vi "RSZVB Set Fixed Power To Signal.vi"(7 "Fixed Power (-25.0)":dbl=-25.0 format="%^.3e", 8 "error in (no error)":errorcluster {"code" format="%.0x"}, 9 "Signal (RF)":i32(ring) items=["RF"=0, "IF"=2, "LO 1"=3, "LO 2"=4, "Aux LO"=5], 10 "Channel (1)":i32=1, 11 "VISA resource name":refnum<visa-resource-name>) -> (0 "error out":errorcluster {"code" format="%.0x"}, 3 "VISA resource name out":refnum<visa-resource-name>)   [LabVIEW 2011]
doc: "This VI assigns a fixed power to the RF, LO 1, LO 2, Aux LO, or to the IF signal.\n\nRemote-control command(s):\nSOURce<Ch>:FREQuency<Pt>:CONVersion:MIXer:PMFixed RF | LO | LO1 | LO2 | AUXLo | IF, <fixed_power>"
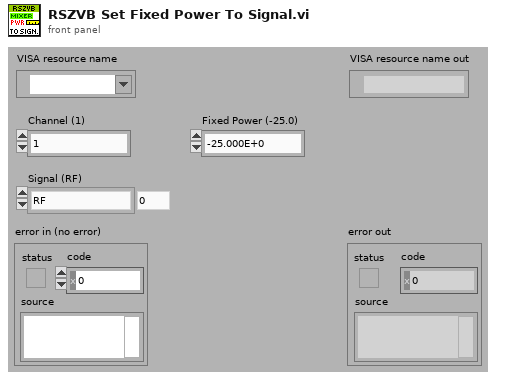
[diagram p1: front panel]
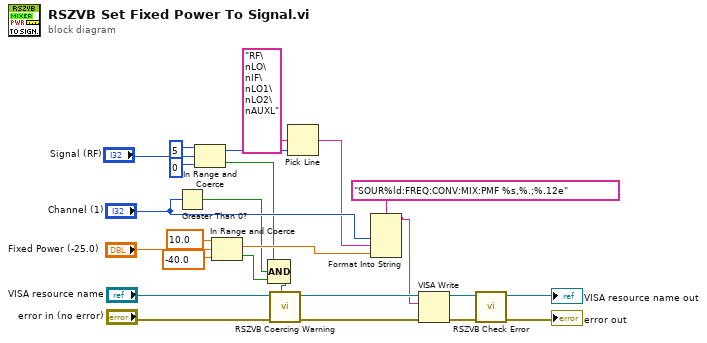
[diagram p0: block diagram]
diagram:
  n1 = Greater Than 0?(x="Channel (1)") -> (x > 0?=w4:bool)
  n2 = In Range and Coerce(upper limit=5, x="Signal (RF)", lower limit=0) -> (coerced(x)=w8:i32, In Range?=w1:bool)
  n3 = In Range and Coerce(upper limit=10.0, x="Fixed Power (-25.0)", lower limit=-40.0) -> (coerced(x)=w13:dbl, In Range?=w12:bool)
  n4 = Compound Arithmetic op=AND(w1, w4, w12) -> (w21:bool)
  n5 = call "RSZVB Coercing Warning.vi"("In Range?"=w21, "error in (no error)"="error in (no error)", "VISA session"="VISA resource name") -> ("error out"=w24:errorcluster, "dup VISA session"=w25:refnum<visa-resource-name>)  [unwired: 7 in]
  n6 = Pick Line(multi-line string="RF\nLO\nIF\nLO1\nLO2\nAUXL", line index=w8) -> (output string=w2:string)  [unwired: 1 in]
  n7 = Format Into String(format string="SOUR%ld:FREQ:CONV:MIX:PMF %s,%.;%.12e", "Channel (1)", w2, w13) -> (resulting string=w17:string)  [unwired: 2 in, 1 out]
  n8 = VISA Write(VISA resource name=w25, write buffer=w17, error in (no error)=w24) -> (VISA resource name out=w22:refnum<visa-resource-name>, error out=w23:errorcluster)  [unwired: 1 out]
  n9 = call "RSZVB Check Error.vi"("error in (no error)"=w23, "VISA session"=w22) -> ("error out"=→"error out":errorcluster, "dup VISA session"=→"VISA resource name out":refnum<visa-resource-name>)  [unwired: 8 in]
